vi "Handle Alerts.vi"(8 "error in (no error)":errorcluster, 11 "[Tags and Alerts]":T1[](array[typedef])) -> (0 "error out":errorcluster)   [LabVIEW 2014]
uses:
  Public Controls/Alert Data.ctl
  RT - Analysis.lvlib
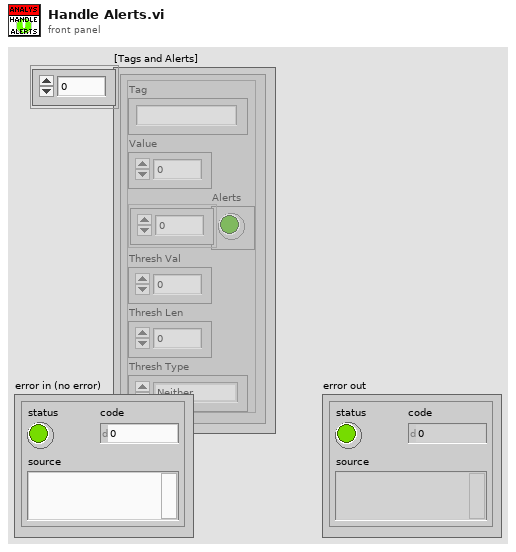
[diagram p1: front panel]
types:
  T1 = typedef "RT - Analysis.lvlib/Alert Data.ctl" = cluster{"Tag":string, "Value":dbl, "Alerts":bool[], "Thresh Val":dbl, "Thresh Len":dbl, "Thresh Type":enum16{"Neither", "Max", "Min"}}
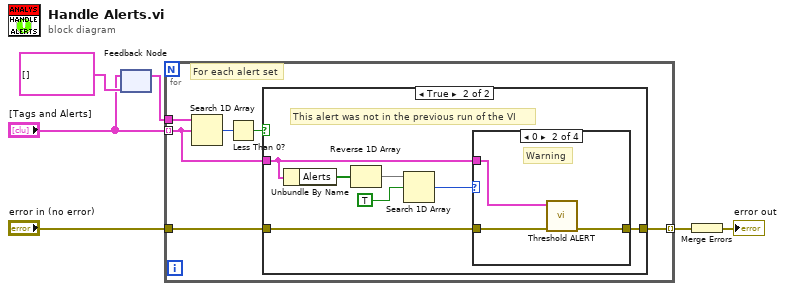
[diagram p0: block diagram]
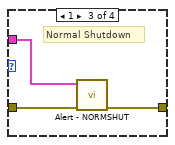
[diagram p4: hidden frame]
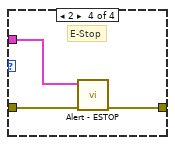
[diagram p5: hidden frame]
diagram:
  n1 = feedback #1(T1[] [] ("[Tags and Alerts]")) -> (w6:T1[])
  n2 = feedback-in #1("[Tags and Alerts]") -> ()
  n3 = for {
    tunnel: [w7] -> w1 mode=indexing
    tunnel: "error in (no error)" -> [w8]
    tunnel: "[Tags and Alerts]" -> [w9] mode=indexing
    tunnel: w6 -> [w12]
    # "For each alert set"
    n4 = Search 1D Array(1D array=w12, element=w9) -> (index of element=w11:i32)  [unwired: 1 in]
    n5 = Less Than 0?(x=w11) -> (x < 0?=w10:bool)
    n6 = case shown="True" w10 {
      tunnel: w9 -> [_ w14]
      tunnel: w8 -> [w13 w15]
      tunnel: [w13 w16] -> w7
      frame False {
      }
      frame True {
        # "This alert was not in the previous run of the VI"
        n7 = Unbundle By Name(w14) -> ("Alerts"=w20:bool[])
        n8 = Reverse 1D Array(array=w20) -> (reversed array=w19:bool[])
        n9 = Search 1D Array(1D array=w19, element=TRUE) -> (index of element=w17:i32)  [unwired: 1 in]
        n10 = case shown="0" w17 {
          tunnel: [w21 w23 w26 w29] -> w16
          tunnel: w15 -> [w21 w24 w27 w30]
          tunnel: w14 -> [_ w22 w25 w28]
          frame Default {
          }
          frame 0 {
            # "Warning"
            n11 = call "Threshold ALERT.vi"("error in (no error)"=w24, "Alert Data"=w22) -> ("error out"=w23:errorcluster)  [unwired: 9 in]
          }
          frame 1 {
            # "Normal Shutdown"
            n12 = call "Alert - NORMSHUT.vi"("error in (no error)"=w27, "Alert Data"=w25) -> ("error out"=w26:errorcluster)  [unwired: 9 in]
          }
          frame 2 {
            # "E-Stop"
            n13 = call "Alert - ESTOP.vi"("error in (no error)"=w30, "Alert Data"=w28) -> ("error out"=w29:errorcluster)  [unwired: 9 in]
          }
        }
      }
    }
  }
  n14 = Merge Errors(w1) -> (→"error out":errorcluster)
